vi "Read Control Values.vi"(8 "error in (no error)":errorcluster, 11 "Control Refnums in":refnum<vi>[](array[refnum])) -> (0 "error out":errorcluster, 1 "Variable Values":dbl[](array[numeric]), 2 "Variable Names":string[](array[string]), 3 "Control Refnums out":refnum<vi>[](array[refnum]))   [LabVIEW 2022 SP3, in "Expressions.lvlib"]
uses:
  Expressions.lvlib
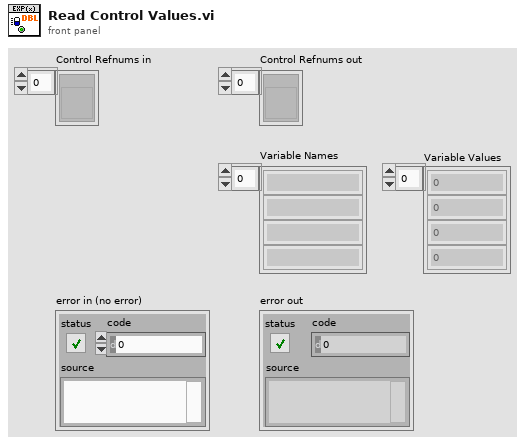
[diagram p1: front panel]
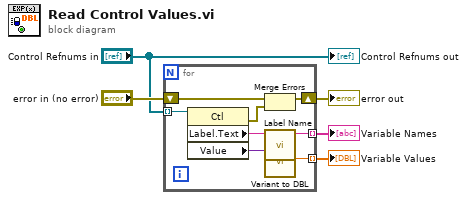
[diagram p0: block diagram]
diagram:
  n1 = for {
    tunnel: "Control Refnums in" -> [w10] mode=indexing
    shift-right: [w12] -> w5
    shift-left: "error in (no error)" -> [w11]
    tunnel: [w7] -> w2 mode=indexing
    tunnel: [w6] -> w1 mode=indexing
    n2 = property class="Ctl"(reference=w10) -> (error out=w13:errorcluster, "Label.Text"=w9:string, "Value"=w8:variant)  [unwired: 1 in, 1 out]
    n3 = Merge Errors(w11, w13) -> (w12:errorcluster)
    n4 = call "Label Name.vi"("Label Text"=w9) -> ("Variable Name"=w7:string)  [unwired: 10 in]
    n5 = call "Variant to DBL.vi"("Variant"=w8) -> ("Value as DBL"=w6:dbl)  [unwired: 9 in, 1 out]
  }
  "error out" <- w5
  "Variable Names" <- w2
  "Variable Values" <- w1
  "Control Refnums out" <- "Control Refnums in"
